vi "CloseAvi.vi"(8 "error in (no error)":errorcluster, 10 "Refnum in Avi":T1, 11 "Refnum in Image":T2) -> (0 "error out":errorcluster)   [LabVIEW 2015]
uses:
  <vilib>/vision/Image Controls.llb/IMAQ Image.ctl
  <vilib>/vision/Avi.llb/IMAQ AVI2 Refnum.ctl
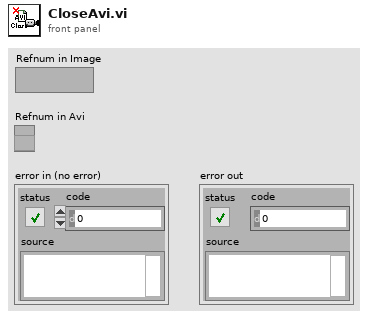
[diagram p1: front panel]
types:
  T1 = typedef "IMAQ AVI2 Refnum.ctl" = refnum<k20>
  T2 = typedef "IMAQ Image.ctl" = refnum<image>
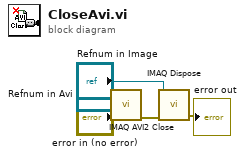
[diagram p0: block diagram]
diagram:
  n1 = call "IMAQ AVI2 Close"("error in (no error)"="error in (no error)", "AVI Refnum"="Refnum in Avi") -> ("error out"=w4:errorcluster)  [unwired: 9 out]
  n2 = call "IMAQ Dispose"("Image"="Refnum in Image", "error in (no error)"=w4) -> ("error out"=→"error out":errorcluster)  [unwired: 1 in, 3 out]
